vi "Permutaciones.vi"(10 "r":i32, 11 "n":i32) -> (3 "n!/(n-r)!":dbl)   [LabVIEW 2020]
doc: "Ayuda a hacer permutaciones para programas a posteriori."
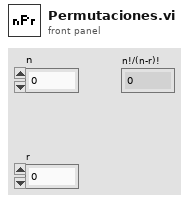
[diagram p1: front panel]
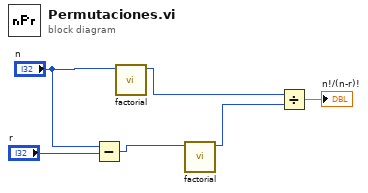
[diagram p0: block diagram]
diagram:
  n1 = Subtract(x="n", y="r") -> (x-y=w4:i32)
  n2 = call "factorial.vi"("n"="n") -> ("n!"=w3:i32)  [unwired: 9 in, 1 out]
  n3 = call "factorial.vi"("n"=w4) -> ("n!"=w2:i32)  [unwired: 9 in, 1 out]
  n4 = Divide(x=w3, y=w2) -> (x/y=→"n!/(n-r)!":dbl)
